vi "Robot Global Data.vi"() -> ()   [LabVIEW 2018]
doc: "This global VI can contain as many global variables as you need. Place a control on the panel, give it a good name. To read or write to it from a VI, drag the icon to the diagram of that VI. You can also drag from the project. Click on the node to change which global you access. You shouldn't have multiple locations writing to a global or it will cause a race-condition."
uses:
  <vilib>/Rock Robotics/WPI/Camera/WPI_CameraImageSize.ctl
  <vilib>/Rock Robotics/WPI/DriverStation/WPI_DriverStationRobotMode2.ctl
  ElevatorAndShift2.ctl
panel:
  in  "Cargo High":bool
  in  "Cargo Mid":bool
  in  "Cargo Low":bool
  in  "Cargo Out":bool
  in  "Decrease Speed":dbl
  in  "Reset Lift Pos":bool
  in  "Hatch  Clamp":bool
  in  "Hatch Push":bool
  out "Wrist encoder pos":i32
  in  "Can Hatch?":bool
  in  "Intake":dbl
  in  "Wrist Pos":dbl
  out "Lift State":T1(ring)
  in  "Hatch Out":bool
  in  "Hatch In":bool
  in  "Cargo Force Out":bool
  in  "Cargo In":bool
  in  "LiftandShift":T2
  in  "Throttle":dbl
  in  "Yaw":dbl
  in  "Robot Mode":T3
  in  "image size":T4=enum."320x240"
  in  "Enable Vision":bool
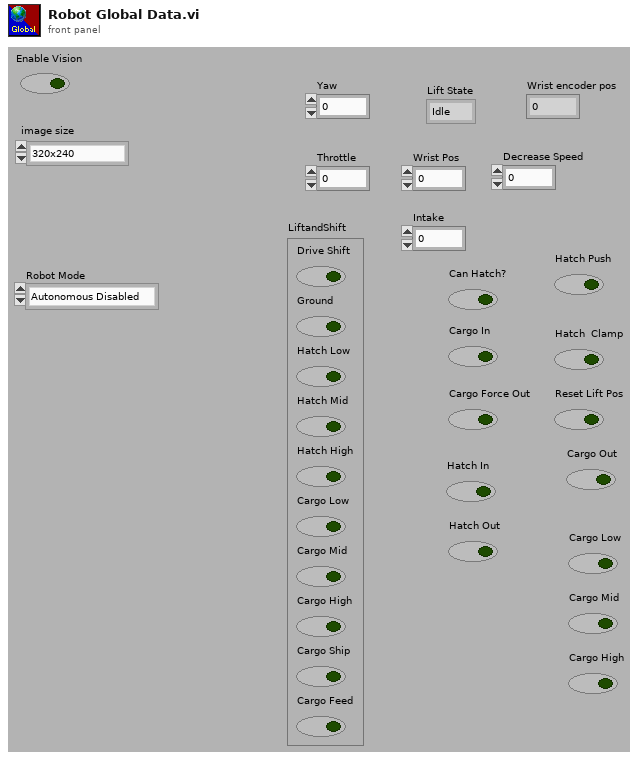
[diagram p1: front panel]
types:
  T1 = enum16{"Idle", "Ground", "Hatch Low", "Hatch Mid", "Hatch High", "Cargo Low", "Cargo Mid", "Cargo High", "Cargo Ship", "Cargo Feed"}
  T2 = typedef "ElevatorAndShift2.ctl" = cluster{"Drive Shift":bool, "Ground":bool, "Hatch Low":bool, "Hatch Mid":bool, "Hatch High":bool, "Cargo Low":bool, "Cargo Mid":bool, "Cargo High":bool, "Cargo Ship":bool, "Cargo Feed":bool}
  T3 = typedef "WPI_DriverStationRobotMode2.ctl" = enum16{"Autonomous Disabled", "Autonomous Enabled", "Teleop Disabled", "Teleop Enabled", "Disconnected", "Finish", "Test Disabled", "Test Enabled", "Emergency Stopped"}
  T4 = typedef "WPI_CameraImageSize.ctl" = enum16{"640x480", "320x240", "160x120", "Custom"}
diagram:
